vi "fgv_sound_q.vi"(7 "cmd":enum16{"create", "write", "read", "close"}(ring), 8 "error in":errorcluster, 11 "data":T1={"FN"=enum."engine", "Data"=variant}) -> (0 "error out":errorcluster, 3 "queue out":refnum<queue>)   [LabVIEW 2019]
uses:
  Ctrl/sound-data.ctl
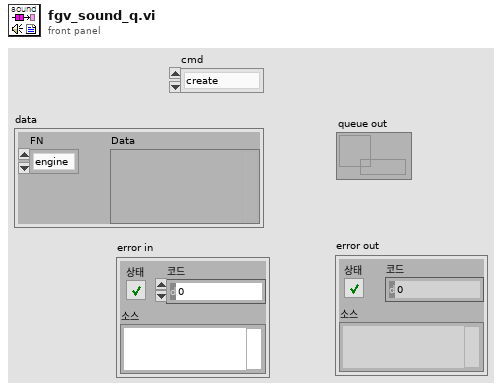
[diagram p1: front panel]
types:
  T1 = typedef "sound-data.ctl" = cluster{"FN":enum16{"check", "unlock", "engine", "warning", "msg", "music"}, "Data":variant}
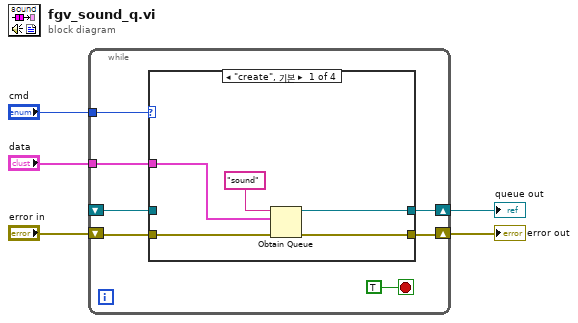
[diagram p0: block diagram]
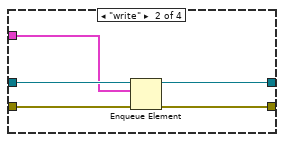
[diagram p2: hidden frame]
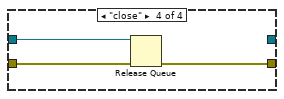
[diagram p4: hidden frame]
diagram:
  n1 = while {
    tunnel: "cmd" -> [w12]
    shift-right: [w8] -> w1
    shift-left: _ -> [w7]
    shift-right: [w9] -> w4
    shift-left: "error in" -> [w10]
    tunnel: "data" -> [w6]
    stop <- TRUE stop-if-true
    n2 = case shown="\"create\", 기본" w12 {
      tunnel: w10 -> [w17 w22 w23 w27]
      tunnel: [w16 w21 w23 w25] -> w9
      tunnel: [w15 w20 w24 _] -> w8
      tunnel: w7 -> [_ w19 w24 w26]
      tunnel: w6 -> [w13 w18 _ _]
      frame "create", Default {
        n3 = Obtain Queue(name (unnamed)="sound" ("이름(이름없음)"), element data type=w13, error in (no error)=w17) -> (queue out=w15:refnum<queue>, error out=w16:errorcluster)  [unwired: 2 in, 1 out]
      }
      frame "write" {
        n4 = Enqueue Element(queue=w19, element=w18, error in (no error)=w22) -> (queue out=w20:refnum<queue>, error out=w21:errorcluster)  [unwired: 1 in, 1 out]
      }
      frame "read" {
      }
      frame "close" {
        n5 = Release Queue(queue=w26, error in (no error)=w27) -> (error out=w25:errorcluster)  [unwired: 1 in, 2 out]
      }
    }
  }
  "error out" <- w4
  "queue out" <- w1
